vi "String to Array Regex.vi"(1 "Regex":string, 2 "Message":string) -> (0 "String to Array":string[](array[string]))   [LabVIEW 2014]
uses:
  <vilib>/regexp/Match Regular Expression.xnode
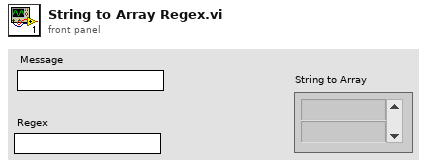
[diagram p1: front panel]
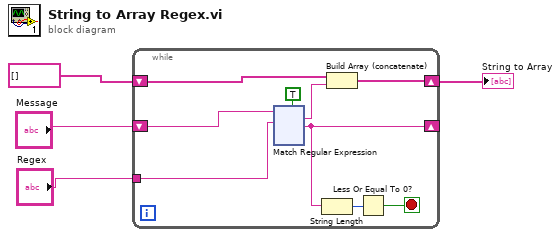
[diagram p0: block diagram]
diagram:
  n1 = while {
    shift-right: [w10] -> _
    shift-left: "Message" -> [w8]
    shift-right: [w6] -> w1
    shift-left: string[] [] -> [w9]
    tunnel: "Regex" -> [w5]
    stop <- w12 stop-if-true
    n2 = xnode "Match Regular Expression"("input string"=w8, "regular expression"=w5, "multiline? (F)"=TRUE) -> ("whole match"=w7:string, "after match"=w10:string)  [unwired: 3 in, 3 out]
    n3 = String Length(string=w10) -> (length=w11:i32)
    n4 = Build Array (concatenate)(w9, w7) -> (w6:string[])
    n5 = Less Or Equal To 0?(x=w11) -> (x <= 0?=w12:bool)
  }
  "String to Array" <- w1
